vi "7.0 Manual Mode Indicators.vi"() -> ()   [LabVIEW 2010]
uses:
  4-High Neurons/4.0-Timing Badass.ctl
  7.0 Manual Mode Display.ctl
  6-OCU Neurons/6.1-UDP Saitek.ctl
  7.0-Global.vi
panel:
  out "Super Heart Beat":T1
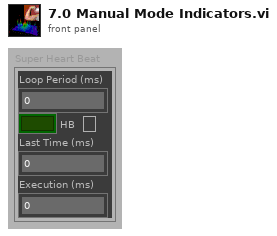
[diagram p1: front panel]
types:
  T1 = typedef "4.0-Timing Badass.ctl" = cluster{"Loop Period (ms)":u32, "HB":bool, "Last Time (ms)":u32, "Execution (ms)":u32}
  T2 = typedef "7.0 Manual Mode Display.ctl" = cluster{"6.1-Saitek Controller":T3, "Time":dbl, "Battery":dbl, "Speed (m/s)":dbl, "Heading":dbl}
  T3 = typedef "6.1-UDP Saitek.ctl" = cluster{"Trig":bool, "2":bool, "3":bool, "4":bool, "5":bool, "6":bool, "7":bool, "8":bool, "9":bool, "10":bool, "11":bool, "Pitch":i32, "Ang":bool[], "Wheel":dbl, "Roll":i32, "Yaw":i32, "Left":i32, "Right":i32}
  T4 = typedef "6.2-Where Reporting.ctl" = cluster{"6.2 GPS Origin":cluster{"Lattitude (dd.mmmmmm)":ext, "Longitude (dd.mmmmmm)":ext}, "6.2 Where Data to Neo-Cortex":cluster{"X (Current)":dbl, "Y (Current) ":dbl, "Heading":dbl, "Steering Angle":dbl}, "6.2 MDF to Neo-Cortex":T5[]}
  T5 = typedef "MDF XY.ctl" = cluster{"Waypoint #":dbl, "X (waypoint)":ext, "Y  (waypoint)":ext, "Vel (desired)":dbl, "Dwell Time":dbl, "Behavior":enum16{"OpenFieldTransit", "WallFollow", "LaneFollow", "ManualMode"}, "Expand1":dbl, "Expand2":dbl, "Expand3":dbl}
  T6 = typedef "6.4-How Reporting Typedef.ctl" = cluster{"Drive Speed (m/s)":dbl, "Lidar Inclination (deg) ":dbl, "Steering Angle (deg)":dbl, "Battery Voltage":dbl, "Drive Encoder Cable Check":bool, "Lidar Drive Encoder Cable Check":bool, "Steer Encoder Cable Check":bool, "Lidar Pos Encoder Cable Check":bool, "Mod Buttons & Blinky Cable Check":bool, "Lidar Data Cable Check":bool, "Drive Motor Cable Check":bool, "Vector Nav Cable Check":bool, "Lidar Drive Cable Check":bool, "Steer Drive Cable Check":bool, "Reverse?":bool, "Steering Control Voltage":dbl, "Drive Control Voltage":dbl, "Lidar Control Voltage":dbl}
  T7 = typedef "6.1-Act.ctl" = cluster{"6.1-Saitek Controller":T3, "Joystick Mode":bool, "Shutdown":bool, "Reset":bool, "Begin":bool}
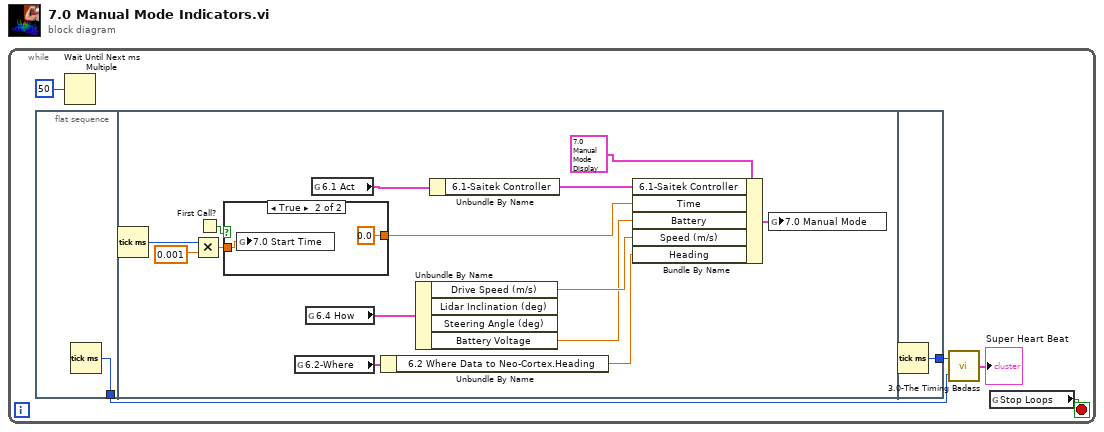
[diagram p0: block diagram]
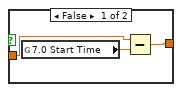
[diagram p2: hidden frame]
diagram:
  n1 = while {
    stop <- w2 stop-if-true
    n2 = flat-sequence {
      tunnel: [w6] -> w4
      tunnel: [w26] -> w5
      frame #0 {
        n3 = Tick Count (ms)() -> (millisecond timer value=w6:u32)
      }
      frame #1 {
        n4 = Tick Count (ms)() -> (millisecond timer value=w11:u32)
        n5 = Multiply(x=w11, y=0.001) -> (x*y=w8:dbl)
        n6 = First Call?() -> (First Call?: T/F=w9:bool)
        n7 = case shown="True" w9 {
          tunnel: w8 -> [w23 w25]
          tunnel: [w21 0.0] -> w7
          frame False {
            n8 = global read "7.0-Global.vi" "7.0 Start Time"() -> (w22:dbl)
            n9 = Subtract(x=w23, y=w22) -> (x-y=w21:dbl)
          }
          frame True {
            n10 = global write "7.0-Global.vi" "7.0 Start Time"(w25) -> ()
          }
        }
        n11 = global read "7.0-Global.vi" "6.2-Where"() -> (w14:T4)
        n12 = global read "7.0-Global.vi" "6.4 How"() -> (w16:T6)
        n13 = global read "7.0-Global.vi" "6.1 Act"() -> (w18:T7)
        n14 = Unbundle By Name(w14) -> ("6.2 Where Data to Neo-Cortex.Heading"=w13:dbl)
        n15 = Unbundle By Name(w16) -> ("Drive Speed (m/s)"=w15:dbl, "Battery Voltage"=w12:dbl)  [unwired: 2 out]
        n16 = Unbundle By Name(w18) -> ("6.1-Saitek Controller"=w17:T3)
        n17 = Bundle By Name(cluster=T2 {"6.1-Saitek Controller"={"Trig"=FALSE, "2"=FALSE, "3"=FALSE, "4"=FALSE, "5"=FALSE, "6"=FALSE, "7"=FALSE, "8"=FALSE, "9"=FALSE, "10"=FALSE, "11"=FALSE, "Pitch"=0, "Ang"=[], "Wheel"=0.0, "Roll"=0, "Yaw"=0, "Left"=0, "Right"=0}, "Time"=0.0, "Battery"=0.0, "Speed (m/s)"=0.0, "Heading"=0.0} ("7.0 Manual Mode"), "6.1-Saitek Controller"=w17, "Time"=w7, "Battery"=w12, "Speed (m/s)"=w15, "Heading"=w13) -> (w20:T2)
        n18 = global write "7.0-Global.vi" "7.0 Manual Mode"(w20) -> ()
      }
      frame #2 {
        n19 = Tick Count (ms)() -> (millisecond timer value=w26:u32)
      }
    }
    n20 = Wait Until Next ms Multiple(millisecond multiple=u32 50) -> ()  [unwired: 1 out]
    n21 = call "3.0-The Timing Badass.vi"("Start"=w4, "End"=w5) -> ("Super Heart Beat"=→"Super Heart Beat":T1)
    n22 = global read "7.0-Global.vi" "Stop Loops"() -> (w2:bool)
  }
